vi "Remove Comments Example.vi"() -> ()   [LabVIEW 2015]
panel:
  out "error out":errorcluster
  in  "error in (no error)":errorcluster
  out "output String":string
  in  "input string":string="{\n\"Cluster\": {\n\"Name\": \"test\", //Give the name of the employee. This is a single line comment\n\"Dept\": \"System Design\" /*Provide the department details. This is a multiple\nline comment*/\n}\n}"
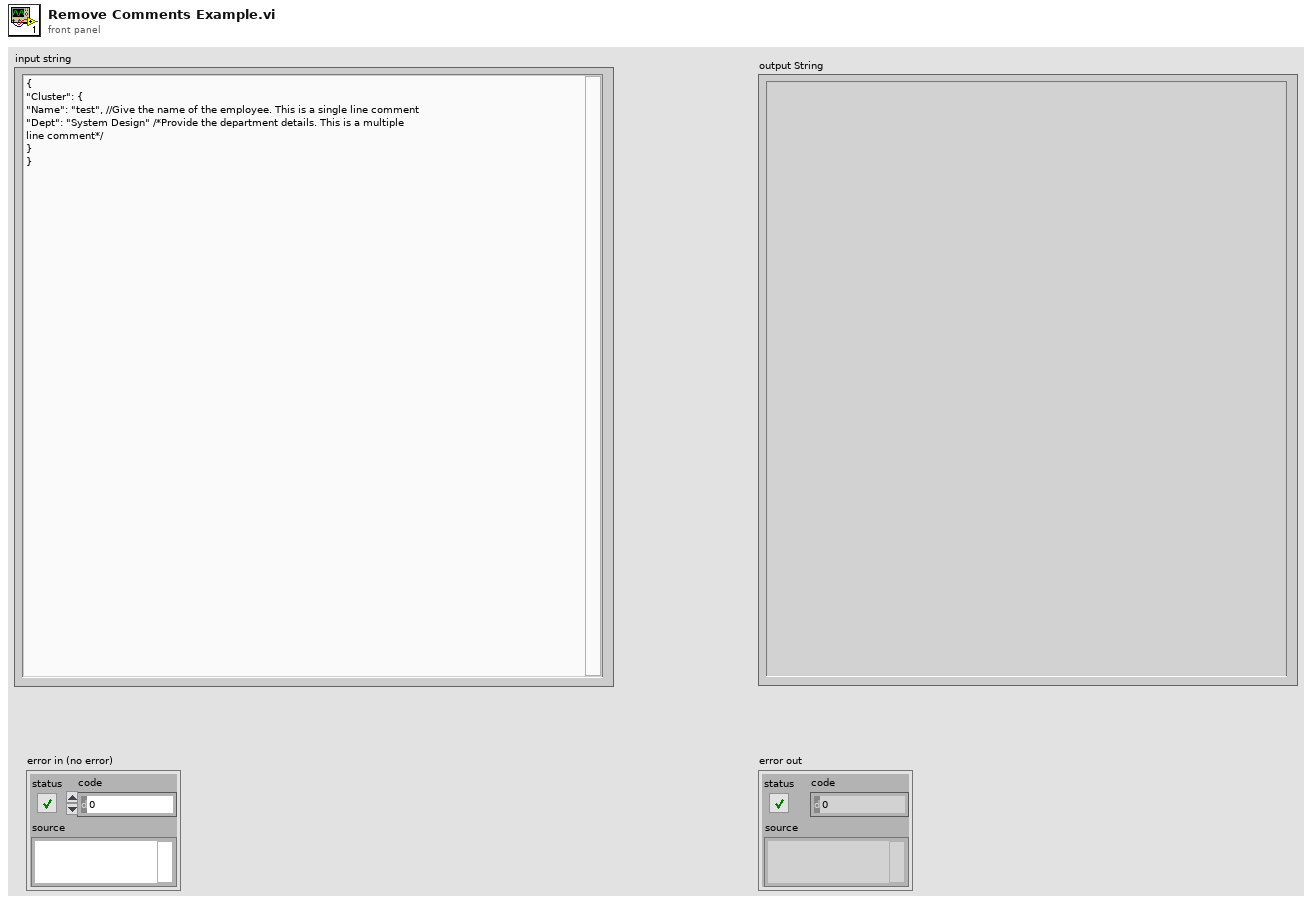
[diagram p1: front panel]
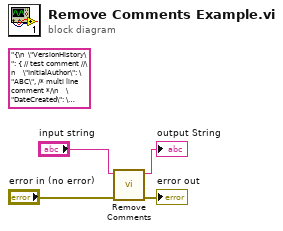
[diagram p0: block diagram]
diagram:
  (unwired) "{\n  \"VersionHistory\": { // test comment //\n    \"InitialAuthor\": \"ABC\", /* multi line comment */\n    \"DateCreated\": \"03:45:56 AM 22/02/2017\", /* multi\nline\ncomment */\n    \"DatesModified\": [ /* multi line * comment */\n      \"03:45:56 AM 22/02/2017\", \n      \"03:45:56 AM 22/02/2017\",\n      \"03:45:56 AM 22/02/2017\"\n    ],\n    \"ModifiedBy\": [\n      \"DEF\",\n      \"GHI\",\n      \"JKL\"\n    ],\n    \"DocumentVersion\": \"2.1.2\",\n    \"ZenParamsSpecVersion\": \"3.2.1\"\n  },\n  \"SystemParameters\": {\n    \"SystemName\": \"Tiger\",\n    \"SystemID\": 123,\n    \"CustomerName\": \"TT\",\n    \"Location\": \"Bangalore\",\n    \"InstallationDate\": \"10-02-2017\",\n    \"NextServiceDate\": \"16-07-2017\",\n    \"ServiceHistory\": [\n      \"16-07-2016\",\n      \"16-08-2016\"\n    ],\n    \"CompatibleZenGage\": \"1.1\",\n    \"TotalNumberOfCameras\": 3,\n    \"NumberOfRacks\": 1,\n    \"SoftwareFeature\": {\n      \"comment_SoftwareFeatures\": \"//Software feature contains controls to Enable/Disable POST, Cp Cpk Report, Analytics, Data Logging and control to set value for Maximum Digital Zoom//\",\n      \"POSTEnable\": true,\n      \"CpCpkReportEnable\": true,\n      \"AnalyticsEnable\": true,\n      \"DataLoggingEnable\": true,\n      \"MaxDigitalZoom\": 5\n    },\n    \"GuideHorizontalPositioningEnable\": true,\n    \"comment_Sensor\": \"//Sensor section contains Name, Unique Id, Controller IO number and Triggering Edge of each sensor//\",\n    \"Sensor\": [\n      {\n        \"Name\": \"pqr\",\n        \"Id\": 1,\n        \"ControllerIONumber\": 12,\n        \"Edge\": \"FALLING\"\n      },\n      {\n        \"Name\": \"stu\",\n        \"Id\": 2,\n        \"ControllerIONumber\": 12,\n        \"Edge\": \"FALLING\"\n      },\n      {\n        \"Name\": \"vwx\",\n        \"Id\": 3,\n        \"ControllerIONumber\": 12,\n        \"Edge\": \"FALLING\"\n      }\n    ],\n    \"comment_Light\": \"//Light section contains Name, Unique Id, Type (Can be Bright field, Dark field, Back light, Front light, Diffuse light, Co-Axial diffuse etc.), Controller IO number and Level (HIGH or LOW) of each Light//\",\n    \"Light\": [\n      {\n        \"Name\": \"Light1\",\n        \"Id\": 1,\n        \"Type\": \"Back\",\n        \"ControllerIONumber\": 23,\n        \"Level\": \"HIGH\"\n      },\n      {\n        \"Name\": \"Light2\",\n        \"Id\": 2,\n        \"Type\": \"Front\",\n        \"ControllerIONumber\": 23,\n        \"Level\": \"HIGH\"\n      },\n      {\n        \"Name\": \"Light3\",\n        \"Id\": 3,\n        \"Type\": \"Back\",\n        \"ControllerIONumber\": 23,\n        \"Level\": \"HIGH\"\n      }\n    ],\n    \"comment_Camera\": \"//Camera section contains Camera Id, Type (Top, Side or Front), Model, Area of Interest (AOI), Trigger Mode, Controller IO Number, Triggering Edge, Pulse Width, Exposure Time in micro seconds, Interface Type (Allowed values are USB3, GigE, USB2), Gain in dB, Calibration details (Date and file path) of each camera//\",\n    \"Camera\": [\n      {\n        \"Id\": 1,\n        \"Type\": \"Top\",\n        \"Model\": \"Basler Ace 5MP\",\n        \"AOI\": [\n          12,\n          34,\n          56,\n          78\n        ],\n        \"TriggerMode\": \"External\",\n        \"ControllerIONumber\": 34,\n        \"Edge\": \"FALLING\",\n        \"PulseWidth\": 233,\n        \"ExposureTimeUSec\": 12,\n        \"InterfaceType\": \"USB3\",\n        \"GainIndB\": 6,\n        \"CalibrationDate\": \"12-01-2017\",\n        \"CalibrationFilePath\": \"C:\\\\Users\\\\veenaj\\\\Desktop\"\n      },\n      {\n        \"Id\": 2,\n        \"Type\": \"Side\",\n        \"Model\": \"Basler Ace 5MP\",\n        \"AOI\": [\n          12,\n          34,\n          56,\n          78\n        ],\n        \"TriggerMode\": \"External\",\n        \"ControllerIONumber\": 34,\n        \"Edge\": \"FALLING\",\n        \"PulseWidth\": 233,\n        \"ExposureTimeUSec\": 12,\n        \"InterfaceType\": \"USB3\",\n        \"GainIndB\": 6,\n        \"CalibrationDate\": \"12/04/17\",\n        \"CalibrationFilePath\": \"C:\\\\Desktop\\\\Calibration\"\n      },\n      {\n        \"Id\": 3,\n        \"Type\": \"Front\",\n        \"Model\": \"Basler Ace 5MP\",\n        \"AOI\": [\n          12,\n          34,\n          56,\n          78\n        ],\n        \"TriggerMode\": \"External\",\n        \"ControllerIONumber\": 34,\n        \"Edge\": \"FALLING\",\n        \"PulseWidth\": 233,\n        \"ExposureTimeUSec\": 12,\n        \"InterfaceType\": \"USB3\",\n        \"GainIndB\": 6,\n        \"CalibrationDate\": \"12/04/17\",\n        \"CalibrationFilePath\": \"C:\\\\Desktop\\\\Calibration\"\n      }\n    ]\n  },\n  \"PartParameters\": {\n    \"comment_PartParameters\": \"//Parts Parameters section includes Number of Parts configured and Parts List. Part List contains Name, Parallel Trigger Threads, Number of measurements and Measurement details//\",\n    \"NumberOfPartsConfigured\": 2,\n    \"PartsList\": [\n      {\n        \"Name\": \"ECU1511\",\n        \"comment_ParallelTriggerThreads\": \"//ParallelTriggerThreads contain Thread Name, Thread Id and Imaging Views. Combination of Camera and Light(s) is defined in Imaging View along with Sensor to Light Delay (in micro seconds), Light to Camera Trigger Delay, Light Pulse Width and Reference Co-ordinate system. Each Imaging View is given a Name and unique ImageId. Camera and Light(s) are accessed by their unique Ids.//\",\n        \"ParallelTriggerThreads\": [\n          {\n            \"ThreadName\": \"TopRack\",\n            \"ThreadId\": 1,\n            \"ImagingViews\": [\n              {\n                \"ImageId\": 1,\n                \"ViewName\": \"TopProfileView\",\n                \"CameraId\": 3,\n                \"LightIds\": [\n                  1,\n                  4,\n                  5\n                ],\n                \"SensorToLightDelayinUSec\": 12,\n                \"LightToCameraTriggerDelay\": 24,\n                \"LightPulseWidth\": 123,\n                \"ReferenceCoordSystem\": {\n                  \"Method\": [\n                    \"A\",\n                    \"B\",\n                    \"C\",\n                    \"D\",\n                    \"R\",\n                    \"V\"\n                  ],\n                  \"comment_RefROI\": \"//Reference ROI is cluster of Left, Top, Right, Bottom and Rotation values//\",\n                  \"ROI1\": [\n                    1014,\n                    95,\n                    1290,\n                    520,\n                    0\n                  ],\n                  \"ROI2\": [\n                    740,\n                    70,\n                    1040,\n                    340,\n                    0\n                  ],\n                  \"ROI3\": [\n                    1060,\n                    88,\n                    723,\n                    85,\n                    0\n                  ],\n                  \"Name\": \"FirstReference\"\n                }\n              },\n              {\n                \"ImageId\": 2,\n                \"ViewName\": \"TopLightView\",\n                \"CameraId\": 2,\n                \"LightIds\": [\n                  2,\n                  3,\n                  5\n                ],\n                \"SensorToLightDelayinUSec\": 12,\n                \"LightToCameraTriggerDelay\": 24,\n                \"LightPulseWidth\": 123,\n                \"ReferenceCoordSystem\": {\n                  \"Method\": [\n                    \"A\",\n                    \"B\",\n                    \"C\",\n                    \"D\",\n                    \"R\",\n                    \"V\"\n                  ],\n                  \"comment_RefROI\": \"//Reference ROI is cluster of Left, Top, Right, Bottom and Rotation values//\",\n                  \"ROI1\": [\n                    1014,\n                    95,\n                    1290,\n                    520,\n                    0\n                  ],\n                  \"ROI2\": [\n                    740,\n                    70,\n                    1040,\n                    340,\n                    0\n                  ],\n                  \"ROI3\": [\n                    1060,\n                    88,\n                    723,\n                    85,\n                    0\n                  ],\n                  \"Name\": \"FirstReference\"\n                }\n              }\n            ]\n          },\n          {\n            \"ThreadName\": \"BottomRack\",\n            \"ThreadId\": 2,\n            \"ImagingViews\": [\n              {\n                \"ImageId\": 1,\n                \"ViewName\": \"TopProfileView\",\n                \"CameraId\": 3,\n                \"LightIds\": [\n                  1,\n                  4,\n                  5\n                ],\n                \"SensorToLightDelayinUSec\": 12,\n                \"LightToCameraTriggerDelay\": 24,\n                \"LightPulseWidth\": 123,\n                \"ReferenceCoordSystem\": {\n                  \"Method\": [\n                    \"A\",\n                    \"B\",\n                    \"C\",\n                    \"D\",\n                    \"R\",\n                    \"V\"\n                  ],\n                  \"comment_RefROI\": \"//Reference ROI is cluster of Left, Top, Right, Bottom and Rotation values//\",\n                  \"ROI1\": [\n                    1014,\n                    95,\n                    1290,\n                    520,\n                    0\n                  ],\n                  \"ROI2\": [\n                    740,\n                    70,\n                    1040,\n                    340,\n                    0\n                  ],\n                  \"ROI3\": [\n                    1060,\n                    88,\n                    723,\n                    85,\n                    0\n                  ],\n                  \"Name\": \"FirstReference\"\n                }\n              },\n              {\n                \"ImageId\": 2,\n                \"ViewName\": \"TopLightView\",\n                \"CameraId\": 2,\n                \"LightIds\": [\n                  2,\n                  3,\n                  5\n                ],\n                \"SensorToLightDelayinUSec\": 12,\n                \"LightToCameraTriggerDelay\": 24,\n                \"LightPulseWidth\": 123,\n                \"ReferenceCoordSystem\": {\n                  \"Method\": [\n                    \"A\",\n                    \"B\",\n                    \"C\",\n                    \"D\",\n                    \"R\",\n                    \"V\"\n                  ],\n                  \"comment_RefROI\": \"//Reference ROI is cluster of Left, Top, Right, Bottom and Rotation values//\",\n                  \"ROI1\": [\n                    1014,\n                    95,\n                    1290,\n                    520,\n                    0\n                  ],\n                  \"ROI2\": [\n                    740,\n                    70,\n                    1040,\n                    340,\n                    0\n                  ],\n                  \"ROI3\": [\n                    1060,\n                    88,\n                    723,\n                    85,\n                    0\n                  ],\n                  \"Name\": \"FirstReference\"\n                }\n              }\n            ]\n          },\n          {\n            \"ThreadName\": \"DentIdentification\",\n            \"ThreadId\": 3,\n            \"ImagingViews\": [\n              {\n                \"ImageId\": 1,\n                \"ViewName\": \"TopProfileView\",\n                \"CameraId\": 3,\n                \"LightIds\": [\n                  1,\n                  4,\n                  5\n                ],\n                \"SensorToLightDelayinUSec\": 12,\n                \"LightToCameraTriggerDelay\": 24,\n                \"LightPulseWidth\": 123,\n                \"ReferenceCoordSystem\": {\n                  \"Method\": [\n                    \"A\",\n                    \"B\",\n                    \"C\",\n                    \"D\",\n                    \"R\",\n                    \"V\"\n                  ],\n                  \"comment_RefROI\": \"//Reference ROI is cluster of Left, Top, Right, Bottom and Rotation values//\",\n                  \"ROI1\": [\n                    23,\n                    78,\n                    99,\n                    25,\n                    0\n                  ],\n                  \"ROI2\": [\n                    67,\n                    97,\n                    43,\n                    9,\n                    0\n                  ],\n                  \"ROI3\": [\n                    45,\n                    88,\n                    723,\n                    85,\n                    0\n                  ],\n                  \"Name\": \"FirstReference\"\n                }\n              }\n            ]\n          }\n        ],\n        \"Number of Measurements\": 3,\n        \"comment_Measurements\": \"//Measurements section contains Name, Type, Enable, Algorithm Sequence, Calibration Co-efficients, User Correction Linearity Coefficients, User Correction Bias Coefficients, LSL, USL, LCL, UCL, Control Limits Violation Threshold, Specification Limits Violation Threshold, Overlay Options, Datalog Enable, Display Icon path for each Measurement//\",\n        \"Measurements\": [\n          {\n            \"Name\": \"CollarWidth\",\n            \"comment_Type\": \"//Type can be Linear or Angle//\",\n            \"Type\": \"Linear\",\n            \"Enable\": true,\n            \"comment_AlgorithmSequence\": \"//Particular Measurement may require sequence of Algorithms. ThreadId and ThreadImageId are mentioned in each Algorithm which corresponds to particular combination of Camera and Light Ids. Result of each Algorithm is stored in a variable and final result is calculated using Math Expression defined.//\",\n            \"AlgorithmSequence\": [\n              {\n                \"AlgoName\": \"MaxClamp\",\n                \"ThreadId\": 1,\n                \"ThreadImageId\": 2,\n                \"Option1\": \"\",\n                \"Option2\": \"\",\n                \"Option3\": \"\",\n                \"LocalRef\": {\n                  \"LocalCoordinateSystemEnable\": true,\n                  \"Method\": [\n                    \"A\",\n                    \"B\",\n                    \"C\",\n                    \"D\",\n                    \"R\",\n                    \"V\"\n                  ],\n                  \"comment_LocalRefROI\": \"//Local Reference ROI is cluster of Left, Top, Right, Bottom and Rotation values//\",\n                  \"ROIs\": [\n                    [\n                      23,\n                      78,\n                      99,\n                      25,\n                      0\n                    ],\n                    [\n                      67,\n                      97,\n                      43,\n                      9,\n                      0\n                    ],\n                    [\n                      45,\n                      88,\n                      723,\n                      85,\n                      0\n                    ]\n                  ],\n                  \"Name\": \"CollarWidthLocalReference\"\n                },\n                \"LocalROIs\": [\n                  [\n                    23,\n                    78,\n                    99,\n                    25,\n                    0\n                  ],\n                  [\n                    67,\n                    97,\n                    43,\n                    9,\n                    0\n                  ],\n                  [\n                    45,\n                    88,\n                    723,\n                    85,\n                    0\n                  ]\n                ],\n                \"comment_Overlay\": \"//OverlayOptions contain Text, Co ordinates, Angle in Degrees, Text Size and Text Color for Overlay//\",\n                \"OverlayOptions\": {\n                  \"OverlayEnable\": true,\n                  \"OverlayText\": \"Collar Width\",\n                  \"OverlayCoords\": [\n                    5,\n                    8\n                  ],\n                  \"OverlayAngle\": 56,\n                  \"OverlayTextSize\": 6,\n                  \"OverlayTextColor\": \"Red\"\n                },\n                \"ResultVariable\": \"M1\"\n              },\n              {\n                \"AlgoName\": \"MoveXYTable\",\n                \"XYDelta\": [\n                  56,\n                  -33.8\n                ]\n              },\n              {\n                \"AlgoName\": \"MaxClamp\",\n                \"ThreadId\": 1,\n                \"ThreadImageId\": 2,\n                \"Option1\": \"\",\n                \"Option2\": \"\",\n                \"Option3\": \"\",\n                \"LocalRef\": {\n                  \"LocalCoordinateSystemEnable\": true,\n                  \"Method\": [\n                    \"A\",\n                    \"B\",\n                    \"C\",\n                    \"D\",\n                    \"R\",\n                    \"V\"\n                  ],\n                  \"ROIs\": [\n                    [\n                      23,\n                      78,\n                      99,\n                      25,\n                      0\n                    ],\n                    [\n                      67,\n                      97,\n                      43,\n                      9,\n                      0\n                    ],\n                    [\n                      45,\n                      88,\n                      723,\n                      85,\n                      0\n                    ]\n                  ],\n                  \"Name\": \"CollarWidthLocalReference\"\n                },\n                \"LocalROIs\": [\n                  [\n                    23,\n                    78,\n                    99,\n                    25,\n                    0\n                  ],\n                  [\n                    67,\n                    97,\n                    43,\n                    9,\n                    0\n                  ],\n                  [\n                    45,\n                    88,\n                    723,\n                    85,\n                    0\n                  ]\n                ],\n                \"comment_Overlay\": \"//OverlayOptions contain Text, Co ordinates, Angle in Degrees, Text Size and Text Color for Overlay//\",\n                \"OverlayOptions\": {\n                  \"OverlayEnable\": true,\n                  \"OverlayText\": \"Collar Width\",\n                  \"OverlayCoords\": [\n                    5,\n                    8\n                  ],\n                  \"OverlayAngle\": 56,\n                  \"OverlayTextSize\": 6,\n                  \"OverlayTextColor\": \"Red\"\n                },\n                \"ResultVariable\": \"M2\"\n              },\n              {\n                \"Algorithm\": \"Math\",\n                \"MathExpression\": \"M2-M1\",\n                \"ResultVariable\": \"M3\"\n              }\n            ],\n            \"CalibrationCoefficients\": [\n              13,\n              8.7,\n              67.9\n            ],\n            \"UserCorrectionLinearityCoeff\": 45,\n            \"UserCorrectionBiasCoeff\": 56,\n            \"comment_LSL\": \"//Lower Specification Limit//\",\n            \"LSL\": 13.5,\n            \"comment_USL\": \"//Upper Specification Limit//\",\n            \"USL\": 15,\n            \"comment_LCL\": \"//Lower Control Limit//\",\n            \"LCL\": 13.5,\n            \"comment_UCL\": \"//Upper Control Limit//\",\n            \"UCL\": 15,\n            \"comment_ControlLimitsViolationThreshold\": \"//If 3 measurement results out of 1000, are crossing LCL and UCL then fail is detected//\",\n            \"ControlLimitsViolationThreshold\": [\n              3,\n              1000\n            ],\n            \"comment_SpecificationLimitsViolationThreshold\": \"//If 5 measurement results out of 5000, are crossing LSL and USL then fail is detected//\",\n            \"SpecificationLimitViolationThreshold\": [\n              5,\n              5000\n            ],\n            \"comment_Overlay\": \"//OverlayOptions contain Text, Co ordinates, Angle in Degrees, Text Size and Text Color for Overlay//\",\n            \"OverlayOptions\": {\n              \"OverlayEnable\": true,\n              \"OverlayText\": \"Collar Width\",\n              \"OverlayCoords\": [\n                5,\n                8\n              ],\n              \"OverlayAngle\": 56,\n              \"OverlayTextSize\": 6,\n              \"OverlayTextColor\": \"Red\"\n            },\n            \"DatalogEnable\": true,\n            \"DisplayIcon\": \"C:\\\\Desktop\\\\displayimage.png\"\n          },\n          {\n            \"Name\": \"Length\",\n            \"comment_Type\": \"//Type can be Linear or Angle//\",\n            \"Type\": \"Linear\",\n            \"Enable\": true,\n            \"comment_AlgorithmSequence\": \"//Particular Measurement may require sequence of Algorithms. ThreadId and ThreadImageId are mentioned in each Algorithm which corresponds to particular combination of Camera and Light Ids. Result of each Algorithm is stored in a variable and final result is calculated using Math Expression defined.//\",\n            \"AlgorithmSequence\": [\n              {\n                \"AlgoName\": \"MaxClamp\",\n                \"ThreadId\": 1,\n                \"ThreadImageId\": 2,\n                \"Option1\": \"\",\n                \"Option2\": \"\",\n                \"Option3\": \"\",\n                \"LocalRef\": {\n                  \"LocalCoordinateSystemEnable\": true,\n                  \"Method\": [\n                    \"A\",\n                    \"B\",\n                    \"C\",\n                    \"D\",\n                    \"R\",\n                    \"V\"\n                  ],\n                  \"comment_LocalRefROI\": \"//Local Reference ROI is cluster of Left, Top, Right, Bottom and Rotation values//\",\n                  \"ROIs\": [\n                    [\n                      23,\n                      78,\n                      99,\n                      25,\n                      0\n                    ],\n                    [\n                      67,\n                      97,\n                      43,\n                      9,\n                      0\n                    ],\n                    [\n                      45,\n                      88,\n                      723,\n                      85,\n                      0\n                    ]\n                  ],\n                  \"Name\": \"CollarWidthLocalReference\"\n                },\n                \"LocalROIs\": [\n                  [\n                    23,\n                    78,\n                    99,\n                    25,\n                    0\n                  ],\n                  [\n                    67,\n                    97,\n                    43,\n                    9,\n                    0\n                  ],\n                  [\n                    45,\n                    88,\n                    723,\n                    85,\n                    0\n                  ]\n                ],\n                \"comment_Overlay\": \"//OverlayOptions contain Text, Co ordinates, Angle in Degrees, Text Size and Text Color for Overlay//\",\n                \"OverlayOptions\": {\n                  \"OverlayEnable\": true,\n                  \"OverlayText\": \"Collar Width\",\n                  \"OverlayCoords\": [\n                    5,\n                    8\n                  ],\n                  \"OverlayAngle\": 56,\n                  \"OverlayTextSize\": 6,\n                  \"OverlayTextColor\": \"Red\"\n                },\n                \"ResultVariable\": \"M1\"\n              },\n              {\n                \"AlgoName\": \"MoveXYTable\",\n                \"XYDelta\": [\n                  56,\n                  -33.8\n                ]\n              },\n              {\n                \"AlgoName\": \"MaxClamp\",\n                \"ThreadId\": 1,\n                \"ThreadImageId\": 2,\n                \"Option1\": \"\",\n                \"Option2\": \"\",\n                \"Option3\": \"\",\n                \"LocalRef\": {\n                  \"LocalCoordinateSystemEnable\": true,\n                  \"Method\": [\n                    \"A\",\n                    \"B\",\n                    \"C\",\n                    \"D\",\n                    \"R\",\n                    \"V\"\n                  ],\n                  \"ROIs\": [\n                    [\n                      23,\n                      78,\n                      99,\n                      25,\n                      0\n                    ],\n                    [\n                      67,\n                      97,\n                      43,\n                      9,\n                      0\n                    ],\n                    [\n                      45,\n                      88,\n                      723,\n                      85,\n                      0\n                    ]\n                  ],\n                  \"Name\": \"CollarWidthLocalReference\"\n                },\n                \"LocalROIs\": [\n                  [\n                    23,\n                    78,\n                    99,\n                    25,\n                    0\n                  ],\n                  [\n                    67,\n                    97,\n                    43,\n                    9,\n                    0\n                  ],\n                  [\n                    45,\n                    88,\n                    723,\n                    85,\n                    0\n                  ]\n                ],\n                \"comment_Overlay\": \"//OverlayOptions contain Text, Co ordinates, Angle in Degrees, Text Size and Text Color for Overlay//\",\n                \"OverlayOptions\": {\n                  \"OverlayEnable\": true,\n                  \"OverlayText\": \"Collar Width\",\n                  \"OverlayCoords\": [\n                    5,\n                    8\n                  ],\n                  \"OverlayAngle\": 56,\n                  \"OverlayTextSize\": 6,\n                  \"OverlayTextColor\": \"Red\"\n                },\n                \"ResultVariable\": \"M2\"\n              },\n              {\n                \"Algorithm\": \"Math\",\n                \"MathExpression\": \"M2-M1\",\n                \"ResultVariable\": \"M3\"\n              }\n            ],\n            \"CalibrationCoefficients\": [\n              13,\n              8.7,\n              67.9\n            ],\n            \"UserCorrectionLinearityCoeff\": 45,\n            \"UserCorrectionBiasCoeff\": 56,\n            \"comment_LSL\": \"//Lower Specification Limit//\",\n            \"LSL\": 13.5,\n            \"comment_USL\": \"//Upper Specification Limit//\",\n            \"USL\": 15,\n            \"comment_LCL\": \"//Lower Control Limit//\",\n            \"LCL\": 13.5,\n            \"comment_UCL\": \"//Upper Control Limit//\",\n            \"UCL\": 15,\n            \"comment_ControlLimitsViolationThreshold\": \"//If 3 measurement results out of 1000, are crossing LCL and UCL then fail is detected//\",\n            \"ControlLimitsViolationThreshold\": [\n              3,\n              1000\n            ],\n            \"comment_SpecificationLimitsViolationThreshold\": \"//If 5 measurement results out of 5000, are crossing LSL and USL then fail is detected//\",\n            \"SpecificationLimitViolationThreshold\": [\n              5,\n              5000\n            ],\n            \"comment_Overlay\": \"//OverlayOptions contain Text, Co ordinates, Angle in Degrees, Text Size and Text Color for Overlay//\",\n            \"OverlayOptions\": {\n              \"OverlayEnable\": true,\n              \"OverlayText\": \"Collar Width\",\n              \"OverlayCoords\": [\n                5,\n                8\n              ],\n              \"OverlayAngle\": 56,\n              \"OverlayTextSize\": 6,\n              \"OverlayTextColor\": \"Red\"\n            },\n            \"DatalogEnable\": true,\n            \"DisplayIcon\": \"C:\\\\Desktop\\\\displayimage.png\"\n          },\n          {\n            \"Name\": \"Length2\",\n            \"comment_Type\": \"//Type can be Linear or Angle//\",\n            \"Type\": \"Linear\",\n            \"Enable\": true,\n            \"comment_AlgorithmSequence\": \"//Particular Measurement may require sequence of Algorithms. ThreadId and ThreadImageId are mentioned in each Algorithm which corresponds to particular combination of Camera and Light Ids. Result of each Algorithm is stored in a variable and final result is calculated using Math Expression defined.//\",\n            \"AlgorithmSequence\": [\n              {\n                \"AlgoName\": \"MaxClamp\",\n                \"ThreadId\": 1,\n                \"ThreadImageId\": 2,\n                \"Option1\": \"\",\n                \"Option2\": \"\",\n                \"Option3\": \"\",\n                \"LocalRef\": {\n                  \"LocalCoordinateSystemEnable\": true,\n                  \"Method\": [\n                    \"A\",\n                    \"B\",\n                    \"C\",\n                    \"D\",\n                    \"R\",\n                    \"V\"\n                  ],\n                  \"comment_LocalRefROI\": \"//Local Reference ROI is cluster of Left, Top, Right, Bottom and Rotation values//\",\n                  \"ROIs\": [\n                    [\n                      23,\n                      78,\n                      99,\n                      25,\n                      0\n                    ],\n                    [\n                      67,\n                      97,\n                      43,\n                      9,\n                      0\n                    ],\n                    [\n                      45,\n                      88,\n                      723,\n                      85,\n                      0\n                    ]\n                  ],\n                  \"Name\": \"CollarWidthLocalReference\"\n                },\n                \"LocalROIs\": [\n                  [\n                    23,\n                    78,\n                    99,\n                    25,\n                    0\n                  ],\n                  [\n                    67,\n                    97,\n                    43,\n                    9,\n                    0\n                  ],\n                  [\n                    45,\n                    88,\n                    723,\n                    85,\n                    0\n                  ]\n                ],\n                \"comment_Overlay\": \"//OverlayOptions contain Text, Co ordinates, Angle in Degrees, Text Size and Text Color for Overlay//\",\n                \"OverlayOptions\": {\n                  \"OverlayEnable\": true,\n                  \"OverlayText\": \"Collar Width\",\n                  \"OverlayCoords\": [\n                    5,\n                    8\n                  ],\n                  \"OverlayAngle\": 56,\n                  \"OverlayTextSize\": 6,\n                  \"OverlayTextColor\": \"Red\"\n                },\n                \"ResultVariable\": \"M1\"\n              },\n              {\n                \"AlgoName\": \"MoveXYTable\",\n                \"XYDelta\": [\n                  56,\n                  -33.8\n                ]\n              },\n              {\n                \"AlgoName\": \"MaxClamp\",\n                \"ThreadId\": 1,\n                \"ThreadImageId\": 2,\n                \"Option1\": \"\",\n                \"Option2\": \"\",\n                \"Option3\": \"\",\n                \"LocalRef\": {\n                  \"LocalCoordinateSystemEnable\": true,\n                  \"Method\": [\n                    \"A\",\n                    \"B\",\n                    \"C\",\n                    \"D\",\n                    \"R\",\n                    \"V\"\n                  ],\n                  \"ROIs\": [\n                    [\n                      23,\n                      78,\n                      99,\n                      25,\n                      0\n                    ],\n                    [\n                      67,\n                      97,\n                      43,\n                      9,\n                      0\n                    ],\n                    [\n                      45,\n                      88,\n                      723,\n                      85,\n                      0\n                    ]\n                  ],\n                  \"Name\": \"CollarWidthLocalReference\"\n                },\n                \"LocalROIs\": [\n                  [\n                    23,\n                    78,\n                    99,\n                    25,\n                    0\n                  ],\n                  [\n                    67,\n                    97,\n                    43,\n                    9,\n                    0\n                  ],\n                  [\n                    45,\n                    88,\n                    723,\n                    85,\n                    0\n                  ]\n                ],\n                \"comment_Overlay\": \"//OverlayOptions contain Text, Co ordinates, Angle in Degrees, Text Size and Text Color for Overlay//\",\n                \"OverlayOptions\": {\n                  \"OverlayEnable\": true,\n                  \"OverlayText\": \"Collar Width\",\n                  \"OverlayCoords\": [\n                    5,\n                    8\n                  ],\n                  \"OverlayAngle\": 56,\n                  \"OverlayTextSize\": 6,\n                  \"OverlayTextColor\": \"Red\"\n                },\n                \"ResultVariable\": \"M2\"\n              },\n              {\n                \"Algorithm\": \"Math\",\n                \"MathExpression\": \"M2-M1\",\n                \"ResultVariable\": \"M3\"\n              }\n            ],\n            \"CalibrationCoefficients\": [\n              13,\n              8.7,\n              67.9\n            ],\n            \"UserCorrectionLinearityCoeff\": 45,\n            \"UserCorrectionBiasCoeff\": 56,\n            \"comment_LSL\": \"//Lower Specification Limit//\",\n            \"LSL\": 13.5,\n            \"comment_USL\": \"//Upper Specification Limit//\",\n            \"USL\": 15,\n            \"comment_LCL\": \"//Lower Control Limit//\",\n            \"LCL\": 13.5,\n            \"comment_UCL\": \"//Upper Control Limit//\",\n            \"UCL\": 15,\n            \"comment_ControlLimitsViolationThreshold\": \"//If 3 measurement results out of 1000, are crossing LCL and UCL then fail is detected//\",\n            \"ControlLimitsViolationThreshold\": [\n              3,\n              1000\n            ],\n            \"comment_SpecificationLimitsViolationThreshold\": \"//If 5 measurement results out of 5000, are crossing LSL and USL then fail is detected//\",\n            \"SpecificationLimitViolationThreshold\": [\n              5,\n              5000\n            ],\n            \"comment_Overlay\": \"//OverlayOptions contain Text, Co ordinates, Angle in Degrees, Text Size and Text Color for Overlay//\",\n            \"OverlayOptions\": {\n              \"OverlayEnable\": true,\n              \"OverlayText\": \"Collar Width\",\n              \"OverlayCoords\": [\n                5,\n                8\n              ],\n              \"OverlayAngle\": 56,\n              \"OverlayTextSize\": 6,\n              \"OverlayTextColor\": \"Red\"\n            },\n            \"DatalogEnable\": true,\n            \"DisplayIcon\": \"C:\\\\Desktop\\\\displayimage.png\"\n          }\n        ]\n      },\n      {\n        \"Name\": \"ECU1512\",\n        \"comment_ParallelTriggerThreads\": \"//ParallelTriggerThreads contain Thread Name, Thread Id and Imaging Views. Combination of Camera and Light(s) is defined in Imaging View along with Sensor to Light Delay (in micro seconds), Light to Camera Trigger Delay, Light Pulse Width and Reference Co-ordinate system. Each Imaging View is given a Name and unique ImageId. Camera and Light(s) are accessed by their unique Ids.//\",\n        \"ParallelTriggerThreads\": [\n          {\n            \"ThreadName\": \"TopRack\",\n            \"ThreadId\": 1,\n            \"ImagingViews\": [\n              {\n                \"ImageId\": 1,\n                \"ViewName\": \"TopProfileView\",\n                \"CameraId\": 3,\n                \"LightIds\": [\n                  1,\n                  4,\n                  5\n                ],\n                \"SensorToLightDelayinUSec\": 12,\n                \"LightToCameraTriggerDelay\": 24,\n                \"LightPulseWidth\": 123,\n                \"ReferenceCoordSystem\": {\n                  \"Method\": [\n                    \"A\",\n                    \"B\",\n                    \"C\",\n                    \"D\",\n                    \"R\",\n                    \"V\"\n                  ],\n                  \"comment_RefROI\": \"//Reference ROI is cluster of Left, Top, Right, Bottom and Rotation values//\",\n                  \"ROI1\": [\n                    1014,\n                    95,\n                    1290,\n                    520,\n                    0\n                  ],\n                  \"ROI2\": [\n                    740,\n                    70,\n                    1040,\n                    340,\n                    0\n                  ],\n                  \"ROI3\": [\n                    1060,\n                    88,\n                    723,\n                    85,\n                    0\n                  ],\n                  \"Name\": \"FirstReference\"\n                }\n              },\n              {\n                \"ImageId\": 2,\n                \"ViewName\": \"TopLightView\",\n                \"CameraId\": 2,\n                \"LightIds\": [\n                  2,\n                  3,\n                  5\n                ],\n                \"SensorToLightDelayinUSec\": 12,\n                \"LightToCameraTriggerDelay\": 24,\n                \"LightPulseWidth\": 123,\n                \"ReferenceCoordSystem\": {\n                  \"Method\": [\n                    \"A\",\n                    \"B\",\n                    \"C\",\n                    \"D\",\n                    \"R\",\n                    \"V\"\n                  ],\n                  \"comment_RefROI\": \"//Reference ROI is cluster of Left, Top, Right, Bottom and Rotation values//\",\n                  \"ROI1\": [\n                    1014,\n                    95,\n                    1290,\n                    520,\n                    0\n                  ],\n                  \"ROI2\": [\n                    740,\n                    70,\n                    1040,\n                    340,\n                    0\n                  ],\n                  \"ROI3\": [\n                    1060,\n                    88,\n                    723,\n                    85,\n                    0\n                  ],\n                  \"Name\": \"FirstReference\"\n                }\n              }\n            ]\n          },\n          {\n            \"ThreadName\": \"BottomRack\",\n            \"ThreadId\": 2,\n            \"ImagingViews\": [\n              {\n                \"ImageId\": 1,\n                \"ViewName\": \"TopProfileView\",\n                \"CameraId\": 3,\n                \"LightIds\": [\n                  1,\n                  4,\n                  5\n                ],\n                \"SensorToLightDelayinUSec\": 12,\n                \"LightToCameraTriggerDelay\": 24,\n                \"LightPulseWidth\": 123,\n                \"ReferenceCoordSystem\": {\n                  \"Method\": [\n                    \"A\",\n                    \"B\",\n                    \"C\",\n                    \"D\",\n                    \"R\",\n                    \"V\"\n                  ],\n                  \"comment_RefROI\": \"//Reference ROI is cluster of Left, Top, Right, Bottom and Rotation values//\",\n                  \"ROI1\": [\n                    1014,\n                    95,\n                    1290,\n                    520,\n                    0\n                  ],\n                  \"ROI2\": [\n                    740,\n                    70,\n                    1040,\n                    340,\n                    0\n                  ],\n                  \"ROI3\": [\n                    1060,\n                    88,\n                    723,\n                    85,\n                    0\n                  ],\n                  \"Name\": \"FirstReference\"\n                }\n              },\n              {\n                \"ImageId\": 2,\n                \"ViewName\": \"TopLightView\",\n                \"CameraId\": 2,\n                \"LightIds\": [\n                  2,\n                  3,\n                  5\n                ],\n                \"SensorToLightDelayinUSec\": 12,\n                \"LightToCameraTriggerDelay\": 24,\n                \"LightPulseWidth\": 123,\n                \"ReferenceCoordSystem\": {\n                  \"Method\": [\n                    \"A\",\n                    \"B\",\n                    \"C\",\n                    \"D\",\n                    \"R\",\n                    \"V\"\n                  ],\n                  \"comment_RefROI\": \"//Reference ROI is cluster of Left, Top, Right, Bottom and Rotation values//\",\n                  \"ROI1\": [\n                    1014,\n                    95,\n                    1290,\n                    520,\n                    0\n                  ],\n                  \"ROI2\": [\n                    740,\n                    70,\n                    1040,\n                    340,\n                    0\n                  ],\n                  \"ROI3\": [\n                    1060,\n                    88,\n                    723,\n                    85,\n                    0\n                  ],\n                  \"Name\": \"FirstReference\"\n                }\n              }\n            ]\n          },\n          {\n            \"ThreadName\": \"DentIdentification\",\n            \"ThreadId\": 3,\n            \"ImagingViews\": [\n              {\n                \"ImageId\": 1,\n                \"ViewName\": \"TopProfileView\",\n                \"CameraId\": 3,\n                \"LightIds\": [\n                  1,\n                  4,\n                  5\n                ],\n                \"SensorToLightDelayinUSec\": 12,\n                \"LightToCameraTriggerDelay\": 24,\n                \"LightPulseWidth\": 123,\n                \"ReferenceCoordSystem\": {\n                  \"Method\": [\n                    \"A\",\n                    \"B\",\n                    \"C\",\n                    \"D\",\n                    \"R\",\n                    \"V\"\n                  ],\n                  \"comment_RefROI\": \"//Reference ROI is cluster of Left, Top, Right, Bottom and Rotation values//\",\n                  \"ROI1\": [\n                    23,\n                    78,\n                    99,\n                    25,\n                    0\n                  ],\n                  \"ROI2\": [\n                    67,\n                    97,\n                    43,\n                    9,\n                    0\n                  ],\n                  \"ROI3\": [\n                    45,\n                    88,\n                    723,\n                    85,\n                    0\n                  ],\n                  \"Name\": \"FirstReference\"\n                }\n              }\n            ]\n          }\n        ],\n        \"comment_Measurements\": \"//Measurements section contains Name, Type, Enable, Algorithm Sequence, Calibration Co-efficients, User Correction Linearity Coefficients, User Correction Bias Coefficients, LSL, USL, LCL, UCL, Control Limits Violation Threshold, Specification Limits Violation Threshold, Overlay Options, Datalog Enable, Display Icon path for each Measurement//\",\n        \"Measurements\": [\n          {\n            \"Name\": \"CollarWidth\",\n            \"comment_Type\": \"//Type can be Linear or Angle//\",\n            \"Type\": \"Linear\",\n            \"Enable\": true,\n            \"comment_AlgorithmSequence\": \"//Particular Measurement may require sequence of Algorithms. ThreadId and ThreadImageId are mentioned in each Algorithm which corresponds to particular combination of Camera and Light Ids. Result of each Algorithm is stored in a variable and final result is calculated using Math Expression defined.//\",\n            \"AlgorithmSequence\": [\n              {\n                \"AlgoName\": \"MaxClamp\",\n                \"ThreadId\": 1,\n                \"ThreadImageId\": 2,\n                \"Option1\": \"\",\n                \"Option2\": \"\",\n                \"Option3\": \"\",\n                \"LocalRef\": {\n                  \"LocalCoordinateSystemEnable\": true,\n                  \"Method\": [\n                    \"A\",\n                    \"B\",\n                    \"C\",\n                    \"D\",\n                    \"R\",\n                    \"V\"\n                  ],\n                  \"comment_LocalRefROI\": \"//Local Reference ROI is cluster of Left, Top, Right, Bottom and Rotation values//\",\n                  \"ROIs\": [\n                    [\n                      23,\n                      78,\n                      99,\n                      25,\n                      0\n                    ],\n                    [\n                      67,\n                      97,\n                      43,\n                      9,\n                      0\n                    ],\n                    [\n                      45,\n                      88,\n                      723,\n                      85,\n                      0\n                    ]\n                  ],\n                  \"Name\": \"CollarWidthLocalReference\"\n                },\n                \"LocalROIs\": [\n                  [\n                    23,\n                    78,\n                    99,\n                    25,\n                    0\n                  ],\n                  [\n                    67,\n                    97,\n                    43,\n                    9,\n                    0\n                  ],\n                  [\n                    45,\n                    88,\n                    723,\n                    85,\n                    0\n                  ]\n                ],\n                \"comment_Overlay\": \"//OverlayOptions contain Text, Co ordinates, Angle in Degrees, Text Size and Text Color for Overlay//\",\n                \"OverlayOptions\": {\n                  \"OverlayEnable\": true,\n                  \"OverlayText\": \"Collar Width\",\n                  \"OverlayCoords\": [\n                    5,\n                    8\n                  ],\n                  \"OverlayAngle\": 56,\n                  \"OverlayTextSize\": 6,\n                  \"OverlayTextColor\": \"Red\"\n                },\n                \"ResultVariable\": \"M1\"\n              },\n              {\n                \"AlgoName\": \"MoveXYTable\",\n                \"XYDelta\": [\n                  56,\n                  -33.8\n                ]\n              },\n              {\n                \"AlgoName\": \"MaxClamp\",\n                \"ThreadId\": 1,\n                \"ThreadImageId\": 2,\n                \"Option1\": \"\",\n                \"Option2\": \"\",\n                \"Option3\": \"\",\n                \"LocalRef\": {\n                  \"LocalCoordinateSystemEnable\": true,\n                  \"Method\": [\n                    \"A\",\n                    \"B\",\n                    \"C\",\n                    \"D\",\n                    \"R\",\n                    \"V\"\n                  ],\n                  \"ROIs\": [\n                    [\n                      23,\n                      78,\n                      99,\n                      25,\n                      0\n                    ],\n                    [\n                      67,\n                      97,\n                      43,\n                      9,\n                      0\n                    ],\n                    [\n                      45,\n                      88,\n                      723,\n                      85,\n                      0\n                    ]\n                  ],\n                  \"Name\": \"CollarWidthLocalReference\"\n                },\n                \"LocalROIs\": [\n                  [\n                    23,\n                    78,\n                    99,\n                    25,\n                    0\n                  ],\n                  [\n                    67,\n                    97,\n                    43,\n                    9,\n                    0\n                  ],\n                  [\n                    45,\n                    88,\n                    723,\n                    85,\n                    0\n                  ]\n                ],\n                \"comment_Overlay\": \"//OverlayOptions contain Text, Co ordinates, Angle in Degrees, Text Size and Text Color for Overlay//\",\n                \"OverlayOptions\": {\n                  \"OverlayEnable\": true,\n                  \"OverlayText\": \"Collar Width\",\n                  \"OverlayCoords\": [\n                    5,\n                    8\n                  ],\n                  \"OverlayAngle\": 56,\n                  \"OverlayTextSize\": 6,\n                  \"OverlayTextColor\": \"Red\"\n                },\n                \"ResultVariable\": \"M2\"\n              },\n              {\n                \"Algorithm\": \"Math\",\n                \"MathExpression\": \"M2-M1\",\n                \"ResultVariable\": \"M3\"\n              }\n            ],\n            \"CalibrationCoefficients\": [\n              13,\n              8.7,\n              67.9\n            ],\n            \"UserCorrectionLinearityCoeff\": 45,\n            \"UserCorrectionBiasCoeff\": 56,\n            \"comment_LSL\": \"//Lower Specification Limit//\",\n            \"LSL\": 13.5,\n            \"comment_USL\": \"//Upper Specification Limit//\",\n            \"USL\": 15,\n            \"comment_LCL\": \"//Lower Control Limit//\",\n            \"LCL\": 13.5,\n            \"comment_UCL\": \"//Upper Control Limit//\",\n            \"UCL\": 15,\n            \"comment_ControlLimitsViolationThreshold\": \"//If 3 measurement results out of 1000, are crossing LCL and UCL then fail is detected//\",\n            \"ControlLimitsViolationThreshold\": [\n              3,\n              1000\n            ],\n            \"comment_SpecificationLimitsViolationThreshold\": \"//If 5 measurement results out of 5000, are crossing LSL and USL then fail is detected//\",\n            \"SpecificationLimitViolationThreshold\": [\n              5,\n              5000\n            ],\n            \"comment_Overlay\": \"//OverlayOptions contain Text, Co ordinates, Angle in Degrees, Text Size and Text Color for Overlay//\",\n            \"OverlayOptions\": {\n              \"OverlayEnable\": true,\n              \"OverlayText\": \"Collar Width\",\n              \"OverlayCoords\": [\n                5,\n                8\n              ],\n              \"OverlayAngle\": 56,\n              \"OverlayTextSize\": 6,\n              \"OverlayTextColor\": \"Red\"\n            },\n            \"DatalogEnable\": true,\n            \"DisplayIcon\": \"C:\\\\Desktop\\\\displayimage.png\"\n          },\n          {\n            \"Name\": \"Length\",\n            \"comment_Type\": \"//Type can be Linear or Angle//\",\n            \"Type\": \"Linear\",\n            \"Enable\": true,\n            \"comment_AlgorithmSequence\": \"//Particular Measurement may require sequence of Algorithms. ThreadId and ThreadImageId are mentioned in each Algorithm which corresponds to particular combination of Camera and Light Ids. Result of each Algorithm is stored in a variable and final result is calculated using Math Expression defined.//\",\n            \"AlgorithmSequence\": [\n              {\n                \"AlgoName\": \"MaxClamp\",\n                \"ThreadId\": 1,\n                \"ThreadImageId\": 2,\n                \"Option1\": \"\",\n                \"Option2\": \"\",\n                \"Option3\": \"\",\n                \"LocalRef\": {\n                  \"LocalCoordinateSystemEnable\": true,\n                  \"Method\": [\n                    \"A\",\n                    \"B\",\n                    \"C\",\n                    \"D\",\n                    \"R\",\n                    \"V\"\n                  ],\n                  \"comment_LocalRefROI\": \"//Local Reference ROI is cluster of Left, Top, Right, Bottom and Rotation values//\",\n                  \"ROIs\": [\n                    [\n                      23,\n                      78,\n                      99,\n                      25,\n                      0\n                    ],\n                    [\n                      67,\n                      97,\n                      43,\n                      9,\n                      0\n                    ],\n                    [\n                      45,\n                      88,\n                      723,\n                      85,\n                      0\n                    ]\n                  ],\n                  \"Name\": \"CollarWidthLocalReference\"\n                },\n                \"LocalROIs\": [\n                  [\n                    23,\n                    78,\n                    99,\n                    25,\n                    0\n                  ],\n                  [\n                    67,\n                    97,\n                    43,\n                    9,\n                    0\n                  ],\n                  [\n                    45,\n                    88,\n                    723,\n                    85,\n                    0\n                  ]\n                ],\n                \"comment_Overlay\": \"//OverlayOptions contain Text, Co ordinates, Angle in Degrees, Text Size and Text Color for Overlay//\",\n                \"OverlayOptions\": {\n                  \"OverlayEnable\": true,\n                  \"OverlayText\": \"Collar Width\",\n                  \"OverlayCoords\": [\n                    5,\n                    8\n                  ],\n                  \"OverlayAngle\": 56,\n                  \"OverlayTextSize\": 6,\n                  \"OverlayTextColor\": \"Red\"\n                },\n                \"ResultVariable\": \"M1\"\n              },\n              {\n                \"AlgoName\": \"MoveXYTable\",\n                \"XYDelta\": [\n                  56,\n                  -33.8\n                ]\n              },\n              {\n                \"AlgoName\": \"MaxClamp\",\n                \"ThreadId\": 1,\n                \"ThreadImageId\": 2,\n                \"Option1\": \"\",\n                \"Option2\": \"\",\n                \"Option3\": \"\",\n                \"LocalRef\": {\n                  \"LocalCoordinateSystemEnable\": true,\n                  \"Method\": [\n                    \"A\",\n                    \"B\",\n                    \"C\",\n                    \"D\",\n                    \"R\",\n                    \"V\"\n                  ],\n                  \"ROIs\": [\n                    [\n                      23,\n                      78,\n                      99,\n                      25,\n                      0\n                    ],\n                    [\n                      67,\n                      97,\n                      43,\n                      9,\n                      0\n                    ],\n                    [\n                      45,\n                      88,\n                      723,\n                      85,\n                      0\n                    ]\n                  ],\n                  \"Name\": \"CollarWidthLocalReference\"\n                },\n                \"LocalROIs\": [\n                  [\n                    23,\n                    78,\n                    99,\n                    25,\n                    0\n                  ],\n                  [\n                    67,\n                    97,\n                    43,\n                    9,\n                    0\n                  ],\n                  [\n                    45,\n                    88,\n                    723,\n                    85,\n                    0\n                  ]\n                ],\n                \"comment_Overlay\": \"//OverlayOptions contain Text, Co ordinates, Angle in Degrees, Text Size and Text Color for Overlay//\",\n                \"OverlayOptions\": {\n                  \"OverlayEnable\": true,\n                  \"OverlayText\": \"Collar Width\",\n                  \"OverlayCoords\": [\n                    5,\n                    8\n                  ],\n                  \"OverlayAngle\": 56,\n                  \"OverlayTextSize\": 6,\n                  \"OverlayTextColor\": \"Red\"\n                },\n                \"ResultVariable\": \"M2\"\n              },\n              {\n                \"Algorithm\": \"Math\",\n                \"MathExpression\": \"M2-M1\",\n                \"ResultVariable\": \"M3\"\n              }\n            ],\n            \"CalibrationCoefficients\": [\n              13,\n              8.7,\n              67.9\n            ],\n            \"UserCorrectionLinearityCoeff\": 45,\n            \"UserCorrectionBiasCoeff\": 56,\n            \"comment_LSL\": \"//Lower Specification Limit//\",\n            \"LSL\": 13.5,\n            \"comment_USL\": \"//Upper Specification Limit//\",\n            \"USL\": 15,\n            \"comment_LCL\": \"//Lower Control Limit//\",\n            \"LCL\": 13.5,\n            \"comment_UCL\": \"//Upper Control Limit//\",\n            \"UCL\": 15,\n            \"comment_ControlLimitsViolationThreshold\": \"//If 3 measurement results out of 1000, are crossing LCL and UCL then fail is detected//\",\n            \"ControlLimitsViolationThreshold\": [\n              3,\n              1000\n            ],\n            \"comment_SpecificationLimitsViolationThreshold\": \"//If 5 measurement results out of 5000, are crossing LSL and USL then fail is detected//\",\n            \"SpecificationLimitViolationThreshold\": [\n              5,\n              5000\n            ],\n            \"comment_Overlay\": \"//OverlayOptions contain Text, Co ordinates, Angle in Degrees, Text Size and Text Color for Overlay//\",\n            \"OverlayOptions\": {\n              \"OverlayEnable\": true,\n              \"OverlayText\": \"Collar Width\",\n              \"OverlayCoords\": [\n                5,\n                8\n              ],\n              \"OverlayAngle\": 56,\n              \"OverlayTextSize\": 6,\n              \"OverlayTextColor\": \"Red\"\n            },\n            \"DatalogEnable\": true,\n            \"DisplayIcon\": \"C:\\\\Desktop\\\\displayimage.png\"\n          },\n          {\n            \"Name\": \"Length2\",\n            \"comment_Type\": \"//Type can be Linear or Angle//\",\n            \"Type\": \"Linear\",\n            \"Enable\": true,\n            \"comment_AlgorithmSequence\": \"//Particular Measurement may require sequence of Algorithms. ThreadId and ThreadImageId are mentioned in each Algorithm which corresponds to particular combination of Camera and Light Ids. Result of each Algorithm is stored in a variable and final result is calculated using Math Expression defined.//\",\n            \"AlgorithmSequence\": [\n              {\n                \"AlgoName\": \"MaxClamp\",\n                \"ThreadId\": 1,\n                \"ThreadImageId\": 2,\n                \"Option1\": \"\",\n                \"Option2\": \"\",\n                \"Option3\": \"\",\n                \"LocalRef\": {\n                  \"LocalCoordinateSystemEnable\": true,\n                  \"Method\": [\n                    \"A\",\n                    \"B\",\n                    \"C\",\n                    \"D\",\n                    \"R\",\n                    \"V\"\n                  ],\n                  \"comment_LocalRefROI\": \"//Local Reference ROI is cluster of Left, Top, Right, Bottom and Rotation values//\",\n                  \"ROIs\": [\n                    [\n                      23,\n                      78,\n                      99,\n                      25,\n                      0\n                    ],\n                    [\n                      67,\n                      97,\n                      43,\n                      9,\n                      0\n                    ],\n                    [\n                      45,\n                      88,\n                      723,\n                      85,\n                      0\n                    ]\n                  ],\n                  \"Name\": \"CollarWidthLocalReference\"\n                },\n                \"LocalROIs\": [\n                  [\n                    23,\n                    78,\n                    99,\n                    25,\n                    0\n                  ],\n                  [\n                    67,\n                    97,\n                    43,\n                    9,\n                    0\n                  ],\n                  [\n                    45,\n                    88,\n                    723,\n                    85,\n                    0\n                  ]\n                ],\n                \"comment_Overlay\": \"//OverlayOptions contain Text, Co ordinates, Angle in Degrees, Text Size and Text Color for Overlay//\",\n                \"OverlayOptions\": {\n                  \"OverlayEnable\": true,\n                  \"OverlayText\": \"Collar Width\",\n                  \"OverlayCoords\": [\n                    5,\n                    8\n                  ],\n                  \"OverlayAngle\": 56,\n                  \"OverlayTextSize\": 6,\n                  \"OverlayTextColor\": \"Red\"\n                },\n                \"ResultVariable\": \"M1\"\n              },\n              {\n                \"AlgoName\": \"MoveXYTable\",\n                \"XYDelta\": [\n                  56,\n                  -33.8\n                ]\n              },\n              {\n                \"AlgoName\": \"MaxClamp\",\n                \"ThreadId\": 1,\n                \"ThreadImageId\": 2,\n                \"Option1\": \"\",\n                \"Option2\": \"\",\n                \"Option3\": \"\",\n                \"LocalRef\": {\n                  \"LocalCoordinateSystemEnable\": true,\n                  \"Method\": [\n                    \"A\",\n                    \"B\",\n                    \"C\",\n                    \"D\",\n                    \"R\",\n                    \"V\"\n                  ],\n                  \"ROIs\": [\n                    [\n                      23,\n                      78,\n                      99,\n                      25,\n                      0\n                    ],\n                    [\n                      67,\n                      97,\n                      43,\n                      9,\n                      0\n                    ],\n                    [\n                      45,\n                      88,\n                      723,\n                      85,\n                      0\n                    ]\n                  ],\n                  \"Name\": \"CollarWidthLocalReference\"\n                },\n                \"LocalROIs\": [\n                  [\n                    23,\n                    78,\n                    99,\n                    25,\n                    0\n                  ],\n                  [\n                    67,\n                    97,\n                    43,\n                    9,\n                    0\n                  ],\n                  [\n                    45,\n                    88,\n                    723,\n                    85,\n                    0\n                  ]\n                ],\n                \"comment_Overlay\": \"//OverlayOptions contain Text, Co ordinates, Angle in Degrees, Text Size and Text Color for Overlay//\",\n                \"OverlayOptions\": {\n                  \"OverlayEnable\": true,\n                  \"OverlayText\": \"Collar Width\",\n                  \"OverlayCoords\": [\n                    5,\n                    8\n                  ],\n                  \"OverlayAngle\": 56,\n                  \"OverlayTextSize\": 6,\n                  \"OverlayTextColor\": \"Red\"\n                },\n                \"ResultVariable\": \"M2\"\n              },\n              {\n                \"Algorithm\": \"Math\",\n                \"MathExpression\": \"M2-M1\",\n                \"ResultVariable\": \"M3\"\n              }\n            ],\n            \"CalibrationCoefficients\": [\n              13,\n              8.7,\n              67.9\n            ],\n            \"UserCorrectionLinearityCoeff\": 45,\n            \"UserCorrectionBiasCoeff\": 56,\n            \"comment_LSL\": \"//Lower Specification Limit//\",\n            \"LSL\": 13.5,\n            \"comment_USL\": \"//Upper Specification Limit//\",\n            \"USL\": 15,\n            \"comment_LCL\": \"//Lower Control Limit//\",\n            \"LCL\": 13.5,\n            \"comment_UCL\": \"//Upper Control Limit//\",\n            \"UCL\": 15,\n            \"comment_ControlLimitsViolationThreshold\": \"//If 3 measurement results out of 1000, are crossing LCL and UCL then fail is detected//\",\n            \"ControlLimitsViolationThreshold\": [\n              3,\n              1000\n            ],\n            \"comment_SpecificationLimitsViolationThreshold\": \"//If 5 measurement results out of 5000, are crossing LSL and USL then fail is detected//\",\n            \"SpecificationLimitViolationThreshold\": [\n              5,\n              5000\n            ],\n            \"comment_Overlay\": \"//OverlayOptions contain Text, Co ordinates, Angle in Degrees, Text Size and Text Color for Overlay//\",\n            \"OverlayOptions\": {\n              \"OverlayEnable\": true,\n              \"OverlayText\": \"Collar Width\",\n              \"OverlayCoords\": [\n                5,\n                8\n              ],\n              \"OverlayAngle\": 56,\n              \"OverlayTextSize\": 6,\n              \"OverlayTextColor\": \"Red\"\n            },\n            \"DatalogEnable\": true,\n            \"DisplayIcon\": \"C:\\\\Desktop\\\\displayimage.png\"\n          }\n        ]\n      },\n      {\n        \"Name\": \"ECU1513\",\n        \"comment_ParallelTriggerThreads\": \"//ParallelTriggerThreads contain Thread Name, Thread Id and Imaging Views. Combination of Camera and Light(s) is defined in Imaging View along with Sensor to Light Delay (in micro seconds), Light to Camera Trigger Delay, Light Pulse Width and Reference Co-ordinate system. Each Imaging View is given a Name and unique ImageId. Camera and Light(s) are accessed by their unique Ids.//\",\n        \"ParallelTriggerThreads\": [\n          {\n            \"ThreadName\": \"TopRack\",\n            \"ThreadId\": 1,\n            \"ImagingViews\": [\n              {\n                \"ImageId\": 1,\n                \"ViewName\": \"TopProfileView\",\n                \"CameraId\": 3,\n                \"LightIds\": [\n                  1,\n                  4,\n                  5\n                ],\n                \"SensorToLightDelayinUSec\": 12,\n                \"LightToCameraTriggerDelay\": 24,\n                \"LightPulseWidth\": 123,\n                \"ReferenceCoordSystem\": {\n                  \"Method\": [\n                    \"A\",\n                    \"B\",\n                    \"C\",\n                    \"D\",\n                    \"R\",\n                    \"V\"\n                  ],\n                  \"comment_RefROI\": \"//Reference ROI is cluster of Left, Top, Right, Bottom and Rotation values//\",\n                  \"ROI1\": [\n                    1014,\n                    95,\n                    1290,\n                    520,\n                    0\n                  ],\n                  \"ROI2\": [\n                    740,\n                    70,\n                    1040,\n                    340,\n                    0\n                  ],\n                  \"ROI3\": [\n                    1060,\n                    88,\n                    723,\n                    85,\n                    0\n                  ],\n                  \"Name\": \"FirstReference\"\n                }\n              },\n              {\n                \"ImageId\": 2,\n                \"ViewName\": \"TopLightView\",\n                \"CameraId\": 2,\n                \"LightIds\": [\n                  2,\n                  3,\n                  5\n                ],\n                \"SensorToLightDelayinUSec\": 12,\n                \"LightToCameraTriggerDelay\": 24,\n                \"LightPulseWidth\": 123,\n                \"ReferenceCoordSystem\": {\n                  \"Method\": [\n                    \"A\",\n                    \"B\",\n                    \"C\",\n                    \"D\",\n                    \"R\",\n                    \"V\"\n                  ],\n                  \"comment_RefROI\": \"//Reference ROI is cluster of Left, Top, Right, Bottom and Rotation values//\",\n                  \"ROI1\": [\n                    1014,\n                    95,\n                    1290,\n                    520,\n                    0\n                  ],\n                  \"ROI2\": [\n                    740,\n                    70,\n                    1040,\n                    340,\n                    0\n                  ],\n                  \"ROI3\": [\n                    1060,\n                    88,\n                    723,\n                    85,\n                    0\n                  ],\n                  \"Name\": \"FirstReference\"\n                }\n              }\n            ]\n          },\n          {\n            \"ThreadName\": \"BottomRack\",\n            \"ThreadId\": 2,\n            \"ImagingViews\": [\n              {\n                \"ImageId\": 1,\n                \"ViewName\": \"TopProfileView\",\n                \"CameraId\": 3,\n                \"LightIds\": [\n                  1,\n                  4,\n                  5\n                ],\n                \"SensorToLightDelayinUSec\": 12,\n                \"LightToCameraTriggerDelay\": 24,\n                \"LightPulseWidth\": 123,\n                \"ReferenceCoordSystem\": {\n                  \"Method\": [\n                    \"A\",\n                    \"B\",\n                    \"C\",\n                    \"D\",\n                    \"R\",\n                    \"V\"\n                  ],\n                  \"comment_RefROI\": \"//Reference ROI is cluster of Left, Top, Right, Bottom and Rotation values//\",\n                  \"ROI1\": [\n                    1014,\n                    95,\n                    1290,\n                    520,\n                    0\n                  ],\n                  \"ROI2\": [\n                    740,\n                    70,\n                    1040,\n                    340,\n                    0\n                  ],\n                  \"ROI3\": [\n                    1060,\n                    88,\n                    723,\n                    85,\n                    0\n                  ],\n                  \"Name\": \"FirstReference\"\n                }\n              },\n              {\n                \"ImageId\": 2,\n                \"ViewName\": \"TopLightView\",\n                \"CameraId\": 2,\n                \"LightIds\": [\n                  2,\n                  3,\n                  5\n                ],\n                \"SensorToLightDelayinUSec\": 12,\n                \"LightToCameraTriggerDelay\": 24,\n                \"LightPulseWidth\": 123,\n                \"ReferenceCoordSystem\": {\n                  \"Method\": [\n                    \"A\",\n                    \"B\",\n                    \"C\",\n                    \"D\",\n                    \"R\",\n                    \"V\"\n                  ],\n                  \"comment_RefROI\": \"//Reference ROI is cluster of Left, Top, Right, Bottom and Rotation values//\",\n                  \"ROI1\": [\n                    1014,\n                    95,\n                    1290,\n                    520,\n                    0\n                  ],\n                  \"ROI2\": [\n                    740,\n                    70,\n                    1040,\n                    340,\n                    0\n                  ],\n                  \"ROI3\": [\n                    1060,\n                    88,\n                    723,\n                    85,\n                    0\n                  ],\n                  \"Name\": \"FirstReference\"\n                }\n              }\n            ]\n          },\n          {\n            \"ThreadName\": \"DentIdentification\",\n            \"ThreadId\": 3,\n            \"ImagingViews\": [\n              {\n                \"ImageId\": 1,\n                \"ViewName\": \"TopProfileView\",\n                \"CameraId\": 3,\n                \"LightIds\": [\n                  1,\n                  4,\n                  5\n                ],\n                \"SensorToLightDelayinUSec\": 12,\n                \"LightToCameraTriggerDelay\": 24,\n                \"LightPulseWidth\": 123,\n                \"ReferenceCoordSystem\": {\n                  \"Method\": [\n                    \"A\",\n                    \"B\",\n                    \"C\",\n                    \"D\",\n                    \"R\",\n                    \"V\"\n                  ],\n                  \"comment_RefROI\": \"//Reference ROI is cluster of Left, Top, Right, Bottom and Rotation values//\",\n                  \"ROI1\": [\n                    23,\n                    78,\n                    99,\n                    25,\n                    0\n                  ],\n                  \"ROI2\": [\n                    67,\n                    97,\n                    43,\n                    9,\n                    0\n                  ],\n                  \"ROI3\": [\n                    45,\n                    88,\n                    723,\n                    85,\n                    0\n                  ],\n                  \"Name\": \"FirstReference\"\n                }\n              }\n            ]\n          }\n        ],\n        \"Number of Measurements\": 3,\n        \"comment_Measurements\": \"//Measurements section contains Name, Type, Enable, Algorithm Sequence, Calibration Co-efficients, User Correction Linearity Coefficients, User Correction Bias Coefficients, LSL, USL, LCL, UCL, Control Limits Violation Threshold, Specification Limits Violation Threshold, Overlay Options, Datalog Enable, Display Icon path for each Measurement//\",\n        \"Measurements\": [\n          {\n            \"Name\": \"CollarWidth\",\n            \"comment_Type\": \"//Type can be Linear or Angle//\",\n            \"Type\": \"Linear\",\n            \"Enable\": true,\n            \"comment_AlgorithmSequence\": \"//Particular Measurement may require sequence of Algorithms. ThreadId and ThreadImageId are mentioned in each Algorithm which corresponds to particular combination of Camera and Light Ids. Result of each Algorithm is stored in a variable and final result is calculated using Math Expression defined.//\",\n            \"AlgorithmSequence\": [\n              {\n                \"AlgoName\": \"MaxClamp\",\n                \"ThreadId\": 1,\n                \"ThreadImageId\": 2,\n                \"Option1\": \"\",\n                \"Option2\": \"\",\n                \"Option3\": \"\",\n                \"LocalRef\": {\n                  \"LocalCoordinateSystemEnable\": true,\n                  \"Method\": [\n                    \"A\",\n                    \"B\",\n                    \"C\",\n                    \"D\",\n                    \"R\",\n                    \"V\"\n                  ],\n                  \"comment_LocalRefROI\": \"//Local Reference ROI is cluster of Left, Top, Right, Bottom and Rotation values//\",\n                  \"ROIs\": [\n                    [\n                      23,\n                      78,\n                      99,\n                      25,\n                      0\n                    ],\n                    [\n                      67,\n                      97,\n                      43,\n                      9,\n                      0\n                    ],\n                    [\n                      45,\n                      88,\n                      723,\n                      85,\n                      0\n                    ]\n                  ],\n                  \"Name\": \"CollarWidthLocalReference\"\n                },\n                \"LocalROIs\": [\n                  [\n                    23,\n                    78,\n                    99,\n                    25,\n                    0\n                  ],\n                  [\n                    67,\n                    97,\n                    43,\n                    9,\n                    0\n                  ],\n                  [\n                    45,\n                    88,\n                    723,\n                    85,\n                    0\n                  ]\n                ],\n                \"comment_Overlay\": \"//OverlayOptions contain Text, Co ordinates, Angle in Degrees, Text Size and Text Color for Overlay//\",\n                \"OverlayOptions\": {\n                  \"OverlayEnable\": true,\n                  \"OverlayText\": \"Collar Width\",\n                  \"OverlayCoords\": [\n                    5,\n                    8\n                  ],\n                  \"OverlayAngle\": 56,\n                  \"OverlayTextSize\": 6,\n                  \"OverlayTextColor\": \"Red\"\n                },\n                \"ResultVariable\": \"M1\"\n              },\n              {\n                \"AlgoName\": \"MoveXYTable\",\n                \"XYDelta\": [\n                  56,\n                  -33.8\n                ]\n              },\n              {\n                \"AlgoName\": \"MaxClamp\",\n                \"ThreadId\": 1,\n                \"ThreadImageId\": 2,\n                \"Option1\": \"\",\n                \"Option2\": \"\",\n                \"Option3\": \"\",\n                \"LocalRef\": {\n                  \"LocalCoordinateSystemEnable\": true,\n                  \"Method\": [\n                    \"A\",\n                    \"B\",\n                    \"C\",\n                    \"D\",\n                    \"R\",\n                    \"V\"\n                  ],\n                  \"ROIs\": [\n                    [\n                      23,\n                      78,\n                      99,\n                      25,\n                      0\n                    ],\n                    [\n                      67,\n                      97,\n                      43,\n                      9,\n                      0\n                    ],\n                    [\n                      45,\n                      88,\n                      723,\n                      85,\n                      0\n                    ]\n                  ],\n                  \"Name\": \"CollarWidthLocalReference\"\n                },\n                \"LocalROIs\": [\n                  [\n                    23,\n                    78,\n                    99,\n                    25,\n                    0\n                  ],\n                  [\n                    67,\n                    97,\n                    43,\n                    9,\n                    0\n                  ],\n                  [\n                    45,\n                    88,\n                    723,\n                    85,\n                    0\n                  ]\n                ],\n                \"comment_Overlay\": \"//OverlayOptions contain Text, Co ordinates, Angle in Degrees, Text Size and Text Color for Overlay//\",\n                \"OverlayOptions\": {\n                  \"OverlayEnable\": true,\n                  \"OverlayText\": \"Collar Width\",\n                  \"OverlayCoords\": [\n                    5,\n                    8\n                  ],\n                  \"OverlayAngle\": 56,\n                  \"OverlayTextSize\": 6,\n                  \"OverlayTextColor\": \"Red\"\n                },\n                \"ResultVariable\": \"M2\"\n              },\n              {\n                \"Algorithm\": \"Math\",\n                \"MathExpression\": \"M2-M1\",\n                \"ResultVariable\": \"M3\"\n              }\n            ],\n            \"CalibrationCoefficients\": [\n              13,\n              8.7,\n              67.9\n            ],\n            \"UserCorrectionLinearityCoeff\": 45,\n            \"UserCorrectionBiasCoeff\": 56,\n            \"comment_LSL\": \"//Lower Specification Limit//\",\n            \"LSL\": 13.5,\n            \"comment_USL\": \"//Upper Specification Limit//\",\n            \"USL\": 15,\n            \"comment_LCL\": \"//Lower Control Limit//\",\n            \"LCL\": 13.5,\n            \"comment_UCL\": \"//Upper Control Limit//\",\n            \"UCL\": 15,\n            \"comment_ControlLimitsViolationThreshold\": \"//If 3 measurement results out of 1000, are crossing LCL and UCL then fail is detected//\",\n            \"ControlLimitsViolationThreshold\": [\n              3,\n              1000\n            ],\n            \"comment_SpecificationLimitsViolationThreshold\": \"//If 5 measurement results out of 5000, are crossing LSL and USL then fail is detected//\",\n            \"SpecificationLimitViolationThreshold\": [\n              5,\n              5000\n            ],\n            \"comment_Overlay\": \"//OverlayOptions contain Text, Co ordinates, Angle in Degrees, Text Size and Text Color for Overlay//\",\n            \"OverlayOptions\": {\n              \"OverlayEnable\": true,\n              \"OverlayText\": \"Collar Width\",\n              \"OverlayCoords\": [\n                5,\n                8\n              ],\n              \"OverlayAngle\": 56,\n              \"OverlayTextSize\": 6,\n              \"OverlayTextColor\": \"Red\"\n            },\n            \"DatalogEnable\": true,\n            \"DisplayIcon\": \"C:\\\\Desktop\\\\displayimage.png\"\n          },\n          {\n            \"Name\": \"Length\",\n            \"comment_Type\": \"//Type can be Linear or Angle//\",\n            \"Type\": \"Linear\",\n            \"Enable\": true,\n            \"comment_AlgorithmSequence\": \"//Particular Measurement may require sequence of Algorithms. ThreadId and ThreadImageId are mentioned in each Algorithm which corresponds to particular combination of Camera and Light Ids. Result of each Algorithm is stored in a variable and final result is calculated using Math Expression defined.//\",\n            \"AlgorithmSequence\": [\n              {\n                \"AlgoName\": \"MaxClamp\",\n                \"ThreadId\": 1,\n                \"ThreadImageId\": 2,\n                \"Option1\": \"\",\n                \"Option2\": \"\",\n                \"Option3\": \"\",\n                \"LocalRef\": {\n                  \"LocalCoordinateSystemEnable\": true,\n                  \"Method\": [\n                    \"A\",\n                    \"B\",\n                    \"C\",\n                    \"D\",\n                    \"R\",\n                    \"V\"\n                  ],\n                  \"comment_LocalRefROI\": \"//Local Reference ROI is cluster of Left, Top, Right, Bottom and Rotation values//\",\n                  \"ROIs\": [\n                    [\n                      23,\n                      78,\n                      99,\n                      25,\n                      0\n                    ],\n                    [\n                      67,\n                      97,\n                      43,\n                      9,\n                      0\n                    ],\n                    [\n                      45,\n                      88,\n                      723,\n                      85,\n                      0\n                    ]\n                  ],\n                  \"Name\": \"CollarWidthLocalReference\"\n                },\n                \"LocalROIs\": [\n                  [\n                    23,\n                    78,\n                    99,\n                    25,\n                    0\n                  ],\n                  [\n                    67,\n                    97,\n                    43,\n                    9,\n                    0\n                  ],\n                  [\n                    45,\n                    88,\n                    723,\n                    85,\n                    0\n                  ]\n                ],\n                \"comment_Overlay\": \"//OverlayOptions contain Text, Co ordinates, Angle in Degrees, Text Size and Text Color for Overlay//\",\n                \"OverlayOptions\": {\n                  \"OverlayEnable\": true,\n                  \"OverlayText\": \"Collar Width\",\n                  \"OverlayCoords\": [\n                    5,\n                    8\n                  ],\n                  \"OverlayAngle\": 56,\n                  \"OverlayTextSize\": 6,\n                  \"OverlayTextColor\": \"Red\"\n                },\n                \"ResultVariable\": \"M1\"\n              },\n              {\n                \"AlgoName\": \"MoveXYTable\",\n                \"XYDelta\": [\n                  56,\n                  -33.8\n                ]\n              },\n              {\n                \"AlgoName\": \"MaxClamp\",\n                \"ThreadId\": 1,\n                \"ThreadImageId\": 2,\n                \"Option1\": \"\",\n                \"Option2\": \"\",\n                \"Option3\": \"\",\n                \"LocalRef\": {\n                  \"LocalCoordinateSystemEnable\": true,\n                  \"Method\": [\n                    \"A\",\n                    \"B\",\n                    \"C\",\n                    \"D\",\n                    \"R\",\n                    \"V\"\n                  ],\n                  \"ROIs\": [\n                    [\n                      23,\n                      78,\n                      99,\n                      25,\n                      0\n                    ],\n                    [\n                      67,\n                      97,\n                      43,\n                      9,\n                      0\n                    ],\n                    [\n                      45,\n                      88,\n                      723,\n                      85,\n                      0\n                    ]\n                  ],\n                  \"Name\": \"CollarWidthLocalReference\"\n                },\n                \"LocalROIs\": [\n                  [\n                    23,\n                    78,\n                    99,\n                    25,\n                    0\n                  ],\n                  [\n                    67,\n                    97,\n                    43,\n                    9,\n                    0\n                  ],\n                  [\n                    45,\n                    88,\n                    723,\n                    85,\n                    0\n                  ]\n                ],\n                \"comment_Overlay\": \"//OverlayOptions contain Text, Co ordinates, Angle in Degrees, Text Size and Text Color for Overlay//\",\n                \"OverlayOptions\": {\n                  \"OverlayEnable\": true,\n                  \"OverlayText\": \"Collar Width\",\n                  \"OverlayCoords\": [\n                    5,\n                    8\n                  ],\n                  \"OverlayAngle\": 56,\n                  \"OverlayTextSize\": 6,\n                  \"OverlayTextColor\": \"Red\"\n                },\n                \"ResultVariable\": \"M2\"\n              },\n              {\n                \"Algorithm\": \"Math\",\n                \"MathExpression\": \"M2-M1\",\n                \"ResultVariable\": \"M3\"\n              }\n            ],\n            \"CalibrationCoefficients\": [\n              13,\n              8.7,\n              67.9\n            ],\n            \"UserCorrectionLinearityCoeff\": 45,\n            \"UserCorrectionBiasCoeff\": 56,\n            \"comment_LSL\": \"//Lower Specification Limit//\",\n            \"LSL\": 13.5,\n            \"comment_USL\": \"//Upper Specification Limit//\",\n            \"USL\": 15,\n            \"comment_LCL\": \"//Lower Control Limit//\",\n            \"LCL\": 13.5,\n            \"comment_UCL\": \"//Upper Control Limit//\",\n            \"UCL\": 15,\n            \"comment_ControlLimitsViolationThreshold\": \"//If 3 measurement results out of 1000, are crossing LCL and UCL then fail is detected//\",\n            \"ControlLimitsViolationThreshold\": [\n              3,\n              1000\n            ],\n            \"comment_SpecificationLimitsViolationThreshold\": \"//If 5 measurement results out of 5000, are crossing LSL and USL then fail is detected//\",\n            \"SpecificationLimitViolationThreshold\": [\n              5,\n              5000\n            ],\n            \"comment_Overlay\": \"//OverlayOptions contain Text, Co ordinates, Angle in Degrees, Text Size and Text Color for Overlay//\",\n            \"OverlayOptions\": {\n              \"OverlayEnable\": true,\n              \"OverlayText\": \"Collar Width\",\n              \"OverlayCoords\": [\n                5,\n                8\n              ],\n              \"OverlayAngle\": 56,\n              \"OverlayTextSize\": 6,\n              \"OverlayTextColor\": \"Red\"\n            },\n            \"DatalogEnable\": true,\n            \"DisplayIcon\": \"C:\\\\Desktop\\\\displayimage.png\"\n          },\n          {\n            \"Name\": \"Length2\",\n            \"comment_Type\": \"//Type can be Linear or Angle//\",\n            \"Type\": \"Linear\",\n            \"Enable\": true,\n            \"comment_AlgorithmSequence\": \"//Particular Measurement may require sequence of Algorithms. ThreadId and ThreadImageId are mentioned in each Algorithm which corresponds to particular combination of Camera and Light Ids. Result of each Algorithm is stored in a variable and final result is calculated using Math Expression defined.//\",\n            \"AlgorithmSequence\": [\n              {\n                \"AlgoName\": \"MaxClamp\",\n                \"ThreadId\": 1,\n                \"ThreadImageId\": 2,\n                \"Option1\": \"\",\n                \"Option2\": \"\",\n                \"Option3\": \"\",\n                \"LocalRef\": {\n                  \"LocalCoordinateSystemEnable\": true,\n                  \"Method\": [\n                    \"A\",\n                    \"B\",\n                    \"C\",\n                    \"D\",\n                    \"R\",\n                    \"V\"\n                  ],\n                  \"comment_LocalRefROI\": \"//Local Reference ROI is cluster of Left, Top, Right, Bottom and Rotation values//\",\n                  \"ROIs\": [\n                    [\n                      23,\n                      78,\n                      99,\n                      25,\n                      0\n                    ],\n                    [\n                      67,\n                      97,\n                      43,\n                      9,\n                      0\n                    ],\n                    [\n                      45,\n                      88,\n                      723,\n                      85,\n                      0\n                    ]\n                  ],\n                  \"Name\": \"CollarWidthLocalReference\"\n                },\n                \"LocalROIs\": [\n                  [\n                    23,\n                    78,\n                    99,\n                    25,\n                    0\n                  ],\n                  [\n                    67,\n                    97,\n                    43,\n                    9,\n                    0\n                  ],\n                  [\n                    45,\n                    88,\n                    723,\n                    85,\n                    0\n                  ]\n                ],\n                \"comment_Overlay\": \"//OverlayOptions contain Text, Co ordinates, Angle in Degrees, Text Size and Text Color for Overlay//\",\n                \"OverlayOptions\": {\n                  \"OverlayEnable\": true,\n                  \"OverlayText\": \"Collar Width\",\n                  \"OverlayCoords\": [\n                    5,\n                    8\n                  ],\n                  \"OverlayAngle\": 56,\n                  \"OverlayTextSize\": 6,\n                  \"OverlayTextColor\": \"Red\"\n                },\n                \"ResultVariable\": \"M1\"\n              },\n              {\n                \"AlgoName\": \"MoveXYTable\",\n                \"XYDelta\": [\n                  56,\n                  -33.8\n                ]\n              },\n              {\n                \"AlgoName\": \"MaxClamp\",\n                \"ThreadId\": 1,\n                \"ThreadImageId\": 2,\n                \"Option1\": \"\",\n                \"Option2\": \"\",\n                \"Option3\": \"\",\n                \"LocalRef\": {\n                  \"LocalCoordinateSystemEnable\": true,\n                  \"Method\": [\n                    \"A\",\n                    \"B\",\n                    \"C\",\n                    \"D\",\n                    \"R\",\n                    \"V\"\n                  ],\n                  \"ROIs\": [\n                    [\n                      23,\n                      78,\n                      99,\n                      25,\n                      0\n                    ],\n                    [\n                      67,\n                      97,\n                      43,\n                      9,\n                      0\n                    ],\n                    [\n                      45,\n                      88,\n                      723,\n                      85,\n                      0\n                    ]\n                  ],\n                  \"Name\": \"CollarWidthLocalReference\"\n                },\n                \"LocalROIs\": [\n                  [\n                    23,\n                    78,\n                    99,\n                    25,\n                    0\n                  ],\n                  [\n                    67,\n                    97,\n                    43,\n                    9,\n                    0\n                  ],\n                  [\n                    45,\n                    88,\n                    723,\n                    85,\n                    0\n                  ]\n                ],\n                \"comment_Overlay\": \"//OverlayOptions contain Text, Co ordinates, Angle in Degrees, Text Size and Text Color for Overlay//\",\n                \"OverlayOptions\": {\n                  \"OverlayEnable\": true,\n                  \"OverlayText\": \"Collar Width\",\n                  \"OverlayCoords\": [\n                    5,\n                    8\n                  ],\n                  \"OverlayAngle\": 56,\n                  \"OverlayTextSize\": 6,\n                  \"OverlayTextColor\": \"Red\"\n                },\n                \"ResultVariable\": \"M2\"\n              },\n              {\n                \"Algorithm\": \"Math\",\n                \"MathExpression\": \"M2-M1\",\n                \"ResultVariable\": \"M3\"\n              }\n            ],\n            \"CalibrationCoefficients\": [\n              13,\n              8.7,\n              67.9\n            ],\n            \"UserCorrectionLinearityCoeff\": 45,\n            \"UserCorrectionBiasCoeff\": 56,\n            \"comment_LSL\": \"//Lower Specification Limit//\",\n            \"LSL\": 13.5,\n            \"comment_USL\": \"//Upper Specification Limit//\",\n            \"USL\": 15,\n            \"comment_LCL\": \"//Lower Control Limit//\",\n            \"LCL\": 13.5,\n            \"comment_UCL\": \"//Upper Control Limit//\",\n            \"UCL\": 15,\n            \"comment_ControlLimitsViolationThreshold\": \"//If 3 measurement results out of 1000, are crossing LCL and UCL then fail is detected//\",\n            \"ControlLimitsViolationThreshold\": [\n              3,\n              1000\n            ],\n            \"comment_SpecificationLimitsViolationThreshold\": \"//If 5 measurement results out of 5000, are crossing LSL and USL then fail is detected//\",\n            \"SpecificationLimitViolationThreshold\": [\n              5,\n              5000\n            ],\n            \"comment_Overlay\": \"//OverlayOptions contain Text, Co ordinates, Angle in Degrees, Text Size and Text Color for Overlay//\",\n            \"OverlayOptions\": {\n              \"OverlayEnable\": true,\n              \"OverlayText\": \"Collar Width\",\n              \"OverlayCoords\": [\n                5,\n                8\n              ],\n              \"OverlayAngle\": 56,\n              \"OverlayTextSize\": 6,\n              \"OverlayTextColor\": \"Red\"\n            },\n            \"DatalogEnable\": true,\n            \"DisplayIcon\": \"C:\\\\Desktop\\\\displayimage.png\"\n          }\n        ]\n      }\n    ]\n  },\n  \"AlgoParameters\": {\n    \"comment_RefROIEdgeOptions\": \"Reference ROI Edge Options is cluster of Edge Polarity, Kernel Size, Width, Minimum Edge Strength, Interpolation Type and Data Processing Method\",\n    \"RefROIEdgeOptions\": [\n      0,\n      2,\n      3,\n      3,\n      50,\n      0\n    ],\n    \"comment_RefROILineOptions\": \"Reference ROI Line Options is cluster of Number of lines, Type, Min. score, Max Score Orientation, Angle Range, Angle Tolerance, Step size, Min. SNR(db), Min Points (%) and Hough Iterations\",\n    \"RefROILineOptions\": [\n      1,\n      1,\n      10,\n      1000,\n      0,\n      10,\n      1,\n      10,\n      0,\n      25\n    ],\n    \"StepSize\": 14\n  },\n  \"ReportParameters\": {},\n  \"DataLogParameters\": {}\n}" ("input string")
  n1 = call "Remove Comments.vi"("error in (no error)"="error in (no error)", "input string"="input string") -> ("error out"=→"error out":errorcluster, "output String"=→"output String":string)  [unwired: 7 in, 1 out]
